vi "Test Report Contain Setup Error Type.vi"(8 "error in (no error)":errorcluster, 11 "XML Report Test in":refnum<class "XML Report Test.lvclass">) -> (0 "error out":errorcluster, 3 "XML Report Test out":refnum<class "XML Report Test.lvclass">)   [LabVIEW 2020, in "XML Report Test.lvclass"]
uses:
  XML Report Test.lvclass
  source/Core/Result/Result.ctl
  source/Core/Result/Status.ctl
  source/Core/Result/Type.ctl
  XML Report Test.lvclass/XML Report Test.ctl
  source/Plugins/XML Report/XML Report.lvclass
  source/Core/Result/Result.lvlib
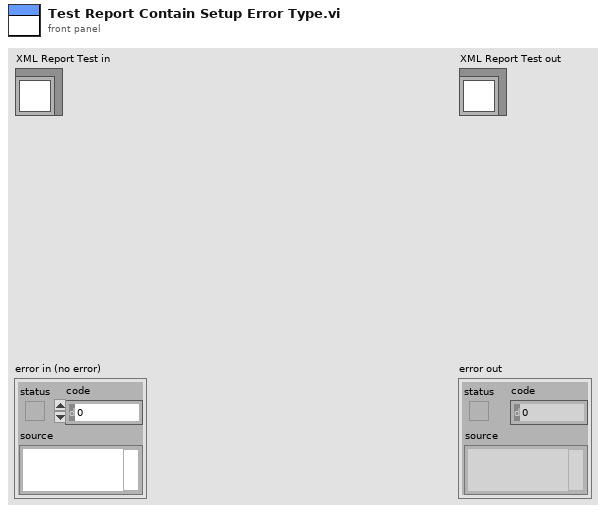
[diagram p1: front panel]
types:
  T1 = typedef "Result.lvlib/Result.ctl" = cluster{"Name":string, "Description":string, "Status":T2, "Result Type":T3, "Execution Time":dbl, "Data":cluster{"Expected":variant, "Actual":variant, "Delta":variant}}
  T2 = typedef "Result.lvlib/Status.ctl" = enum16{"", "Passed", "Failed", "Error", "Skipped", "Setup Error", "Broken", "Teardown Error"}
  T3 = typedef "Result.lvlib/Type.ctl" = enum16{"Test Case", "Test Suite", "Test Run", "Pass", "Fail", "Skip", "Pass if", "Fail if", "Pass if Error", "Fail if Error", "Pass if Equal", "Fail if Equal"}
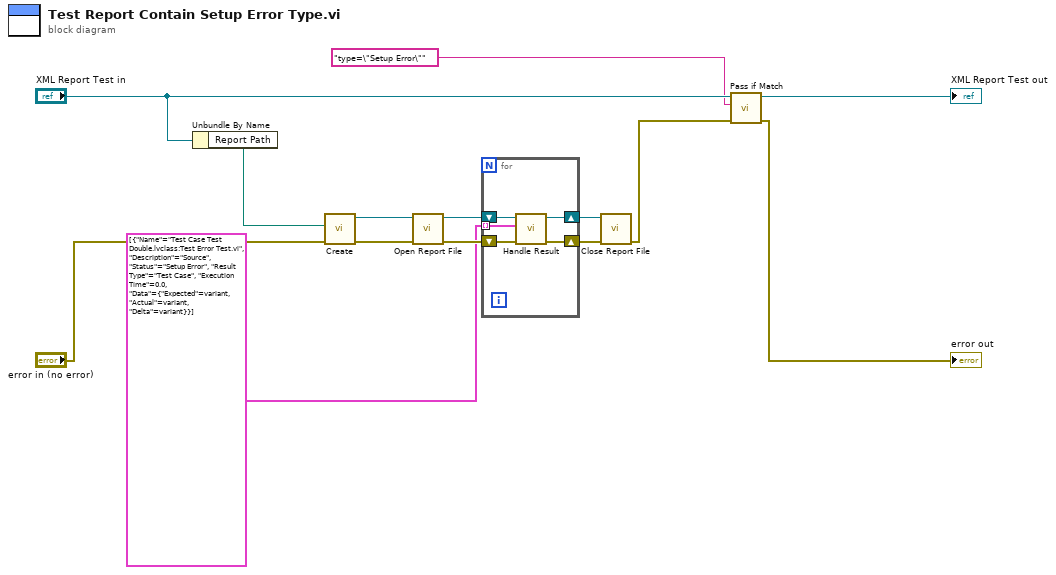
[diagram p0: block diagram]
diagram:
  n1 = Unbundle By Name("XML Report Test in") -> ("Report Path"=w1:path)
  n2 = call "Create.vi"("error in (no error)"="error in (no error)", "Report Path"=w1) -> ("error out"=w3:errorcluster, "XML Report"=w2:refnum<class "XML Report.lvclass">)  [unwired: 8 in]
  n3 = call-dynamic "Open Report File.vi"("error in (no error)"=w3, "XML Report In"=w2) -> ("error out"=w14:errorcluster, "XML Report Out"=w6:refnum<class "XML Report.lvclass">)  [unwired: 8 in]
  n4 = for {
    tunnel: T1[] [{"Name"="Test Case Test Double.lvclass:Test Error Test.vi", "Description"="Source", "Status"=enum."Setup Error", "Result Type"=enum."Test Case", "Execution Time"=0.0, "Data"={"Expected"=variant, "Actual"=variant, "Delta"=variant}}] ("Data") -> [w15] mode=indexing
    shift-right: [w18] -> w7
    shift-left: w14 -> [w19]
    shift-right: [w16] -> w5
    shift-left: w6 -> [w17]
    n5 = call-dynamic "Handle Result.vi"("error in (no error)"=w19, "Result"=w15, "XML Report In"=w17) -> ("error out"=w18:errorcluster, "XML Report Out"=w16:refnum<class "XML Report.lvclass">)  [unwired: 7 in]
  }
  n6 = call-dynamic "Close Report File.vi"("error in (no error)"=w7, "XML Report In"=w5) -> ("error out"=w10:errorcluster)  [unwired: 8 in, 1 out]
  n7 = call "Pass if Match.vi"("error in (no error)"=w10, "regular expression"="type=\"Setup Error\"", "XML Report Test in"="XML Report Test in") -> ("error out"=→"error out":errorcluster, "XML Report Test out"=→"XML Report Test out":refnum<class "XML Report Test.lvclass">)  [unwired: 6 in, 1 out]
